vi "end timer Read.vi"(4 "error in (no error)":errorcluster, 6 "Container State":T4, 7 "Display State In":T1={"Y_State"={"connect"=FALSE, "Y_State"=enum."initialize", "Y"=0.0}, "Write"=FALSE, "button state"=enum."init", "reset_timer"=FALSE, "load_timer"=FALSE, "end_timer"=TRUE}) -> (0 "error out":errorcluster, 2 "Value":bool, 3 "Display State Out":T1={"Y_State"={"connect"=FALSE, "Y_State"=enum."initialize", "Y"=0.0}, "Write"=FALSE, "button state"=enum."init", "reset_timer"=FALSE, "load_timer"=FALSE, "end_timer"=TRUE})   [LabVIEW 2019, in "Heating.lvlib" / "YQ.xctl"]
uses:
  YQ.xctl
  <vilib>/_xctls/Container State.ctl
  State.ctl
  Y_state.ctl
  Y_controlState.ctl
  <vilib>/_xctls/XControlSupport.lvlib
  Heating.lvlib
panel:
  # "Replace the Value Indicator below with an Indicator of desired type.\nDo not remove this Indicator or the others from the connector pane. \nDo not change the connector pane pattern.\nThe Value Indicator should always be the second terminal from top on the output side in the connector pane."
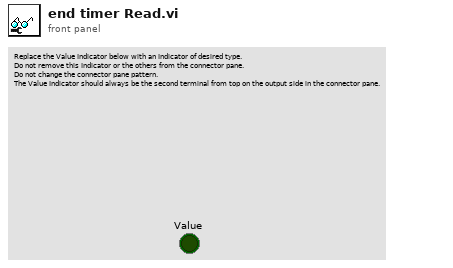
[diagram p1: front panel]
types:
  T1 = typedef "Heating.lvlib/YQ.xctl/State.ctl" = cluster{"Y_State":cluster{"connect":bool, "Y_State":T2, "Y":dbl}, "Write":bool, "button state":T3, "reset_timer":bool, "load_timer":bool, "end_timer":bool}
  T2 = typedef "Heating.lvlib/Y_state.ctl" = enum8{"initialize", "alarm", "min", "stop", "hand", "auto", "max"}
  T3 = typedef "Heating.lvlib/YQ.xctl/Y_controlState.ctl" = enum16{"init", "not connect", "alarm", "min", "stop", "hand", "value change", "auto", "max"}
  T4 = typedef "XControlSupport.lvlib/Container State.ctl" = cluster{"Indicator?":bool, "Run Mode?":bool, " Refnum":refnum<vi>}
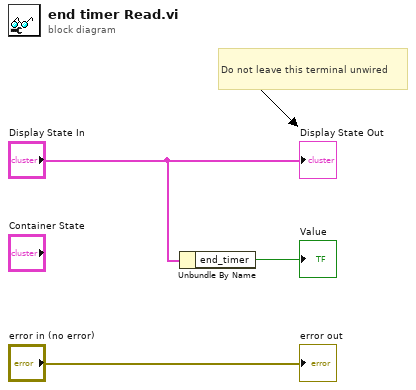
[diagram p0: block diagram]
diagram:
  # "Do not leave this terminal unwired"
  n1 = Unbundle By Name("Display State In") -> ("end_timer"=→"Value":bool)
  "error out" <- "error in (no error)"
  "Display State Out" <- "Display State In"
